vi "GetNextSatae.vi"(4 "Stop2 Switch":T1={"Tag Name"="S060.PXI.Signals.PlltData.SN", "Network Path"="172.15.51.1,1,0", "use opc"=FALSE, "DataSocket Reference"={"CWDSLib._DCWDataSocket"=refnum, "CWDSLib._DCWData"=refnum, "OnDataUpdated"=0, "OnStatusUpdated"=0}} {"DataSocket Reference"."OnStatusUpdated" format="%.0x"; "DataSocket Reference"."OnDataUpdated" format="%.0x"}, 6 "Stop1 Switch":T1={"Tag Name"="S060.PXI.Signals.PlltData.SN", "Network Path"="172.15.51.1,1,0", "use opc"=FALSE, "DataSocket Reference"={"CWDSLib._DCWDataSocket"=refnum, "CWDSLib._DCWData"=refnum, "OnDataUpdated"=0, "OnStatusUpdated"=0}} {"DataSocket Reference"."OnStatusUpdated" format="%.0x"; "DataSocket Reference"."OnDataUpdated" format="%.0x"}, 8 "输入字符串":string, 10 "Done":bool, 11 "debug":bool) -> (3 "after":string)   [LabVIEW 2018]
uses:
  05.UserVI's/type defs/plc path and tag.ctl
  <vilib>/Platform/dataskt.llb/DataSocket Reference Type.ctl
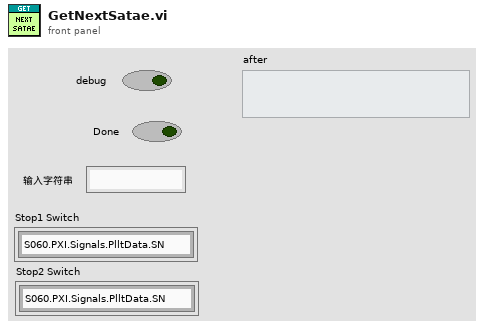
[diagram p1: front panel]
types:
  T1 = typedef "plc path and tag.ctl" = cluster{"Tag Name":string, "Network Path":string, "use opc":bool, "DataSocket Reference":T2}
  T2 = typedef "DataSocket Reference Type.ctl" = cluster{"CWDSLib._DCWDataSocket":refnum<k7>, "CWDSLib._DCWData":refnum<k7>, "OnDataUpdated":u32, "OnStatusUpdated":u32}
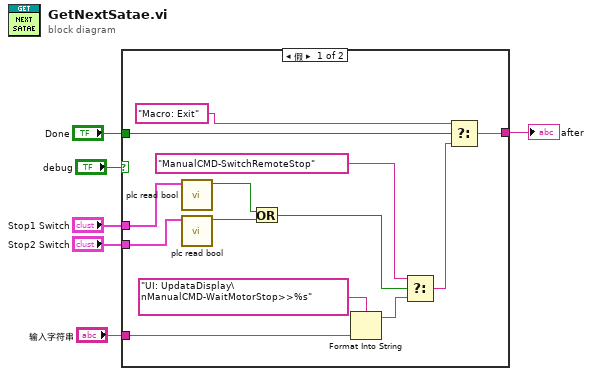
[diagram p0: block diagram]
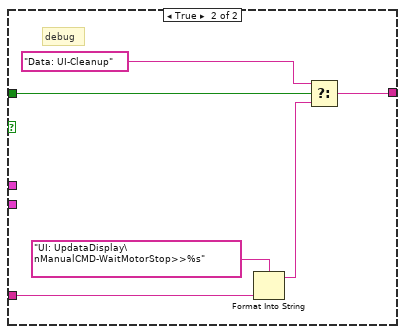
[diagram p2: hidden frame]
diagram:
  n1 = case shown="假" "debug" {
    tunnel: "Done" -> [w16 w22]
    tunnel: [w18 w24] -> w4
    tunnel: "输入字符串" -> [w17 w21]
    tunnel: "Stop2 Switch" -> [w14 _]
    tunnel: "Stop1 Switch" -> [w13 _]
    frame False {
      n2 = call "plc read bool.vi"("addr,tag"=w13) -> ("value"=w11:bool)  [unwired: 9 in, 1 out]
      n3 = call "plc read bool.vi"("addr,tag"=w14) -> ("value"=w12:bool)  [unwired: 9 in, 1 out]
      n4 = Or(x=w11, y=w12) -> (x .or. y?=w10:bool)
      n5 = Format Into String(format string="UI: UpdataDisplay\nManualCMD-WaitMotorStop>>%s", w17) -> (resulting string=w9:string)  [unwired: 2 in, 1 out]
      n6 = Select(t="ManualCMD-SwitchRemoteStop", s=w10, f=w9) -> (s? t:f=w7:string)
      n7 = Select(t="Macro: Exit", s=w16, f=w7) -> (s? t:f=w18:string)
    }
    frame True {
      # "debug"
      n8 = Format Into String(format string="UI: UpdataDisplay\nManualCMD-WaitMotorStop>>%s", w21) -> (resulting string=w20:string)  [unwired: 2 in, 1 out]
      n9 = Select(t="Data: UI-Cleanup", s=w22, f=w20) -> (s? t:f=w24:string)
    }
  }
  "after" <- w4
